vi "Valve_EPICS_Dev4_SSE.vi"() -> ()   [LabVIEW 2014]
uses:
  <userlib>/caLab/Private/Get_PV-1D.vi
  <userlib>/caLab/Private/Put_DBL-1D_PV-1D.vi
panel:
  out "initialized array":i16[](array[numeric])
  in  "stop":bool
  out "sum":i16
  out "0, 1":i16[](array[numeric])
  out "appended array":bool[](array[boolean])
  out "SCL_data":u32[](array[numeric]) caption="data"
  out "SOP_data":u32[](array[numeric]) caption="data"
  out "SCL7":bool
  out "SCL6":bool
  out "SCL5":bool
  out "SCL4":bool
  out "SCL3":bool
  out "SCL2":bool
  out "SCL1":bool
  out "SCL0":bool
  out "SOP7":bool
  out "SOP6":bool
  out "SOP5":bool
  out "SOP4":bool
  out "SOP3":bool
  out "SOP2":bool
  out "SOP1":bool
  out "SOP0":bool
  in  "OPEN7":bool
  in  "OPEN6":bool
  in  "OPEN5":bool
  in  "OPEN4":bool
  in  "OPEN3":bool
  in  "OPEN2":bool
  in  "OPEN1":bool
  in  "OPEN0":bool
  # "Valve control DEV4"
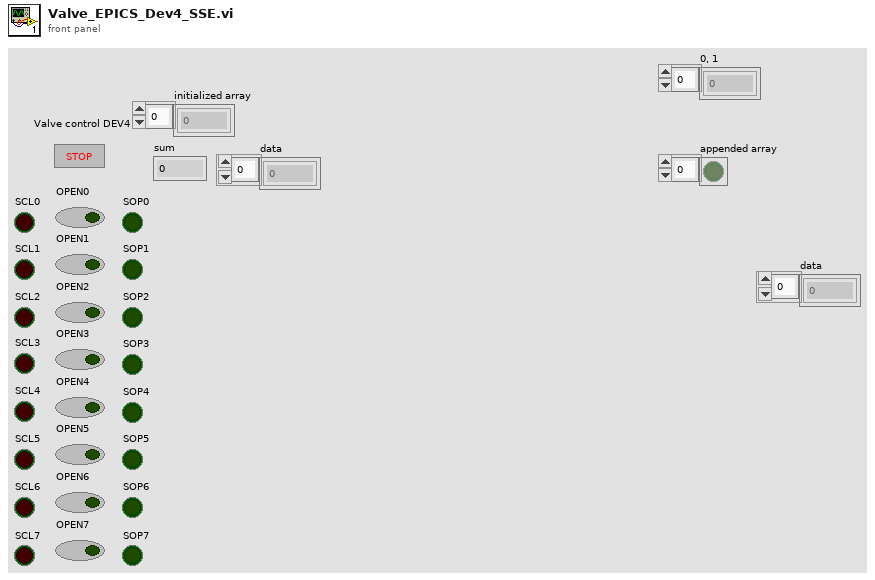
[diagram p1: front panel]
types:
  T1 = typedef "NI_Matrix.lvlib/RealMatrix.ctl" = dbl[][]
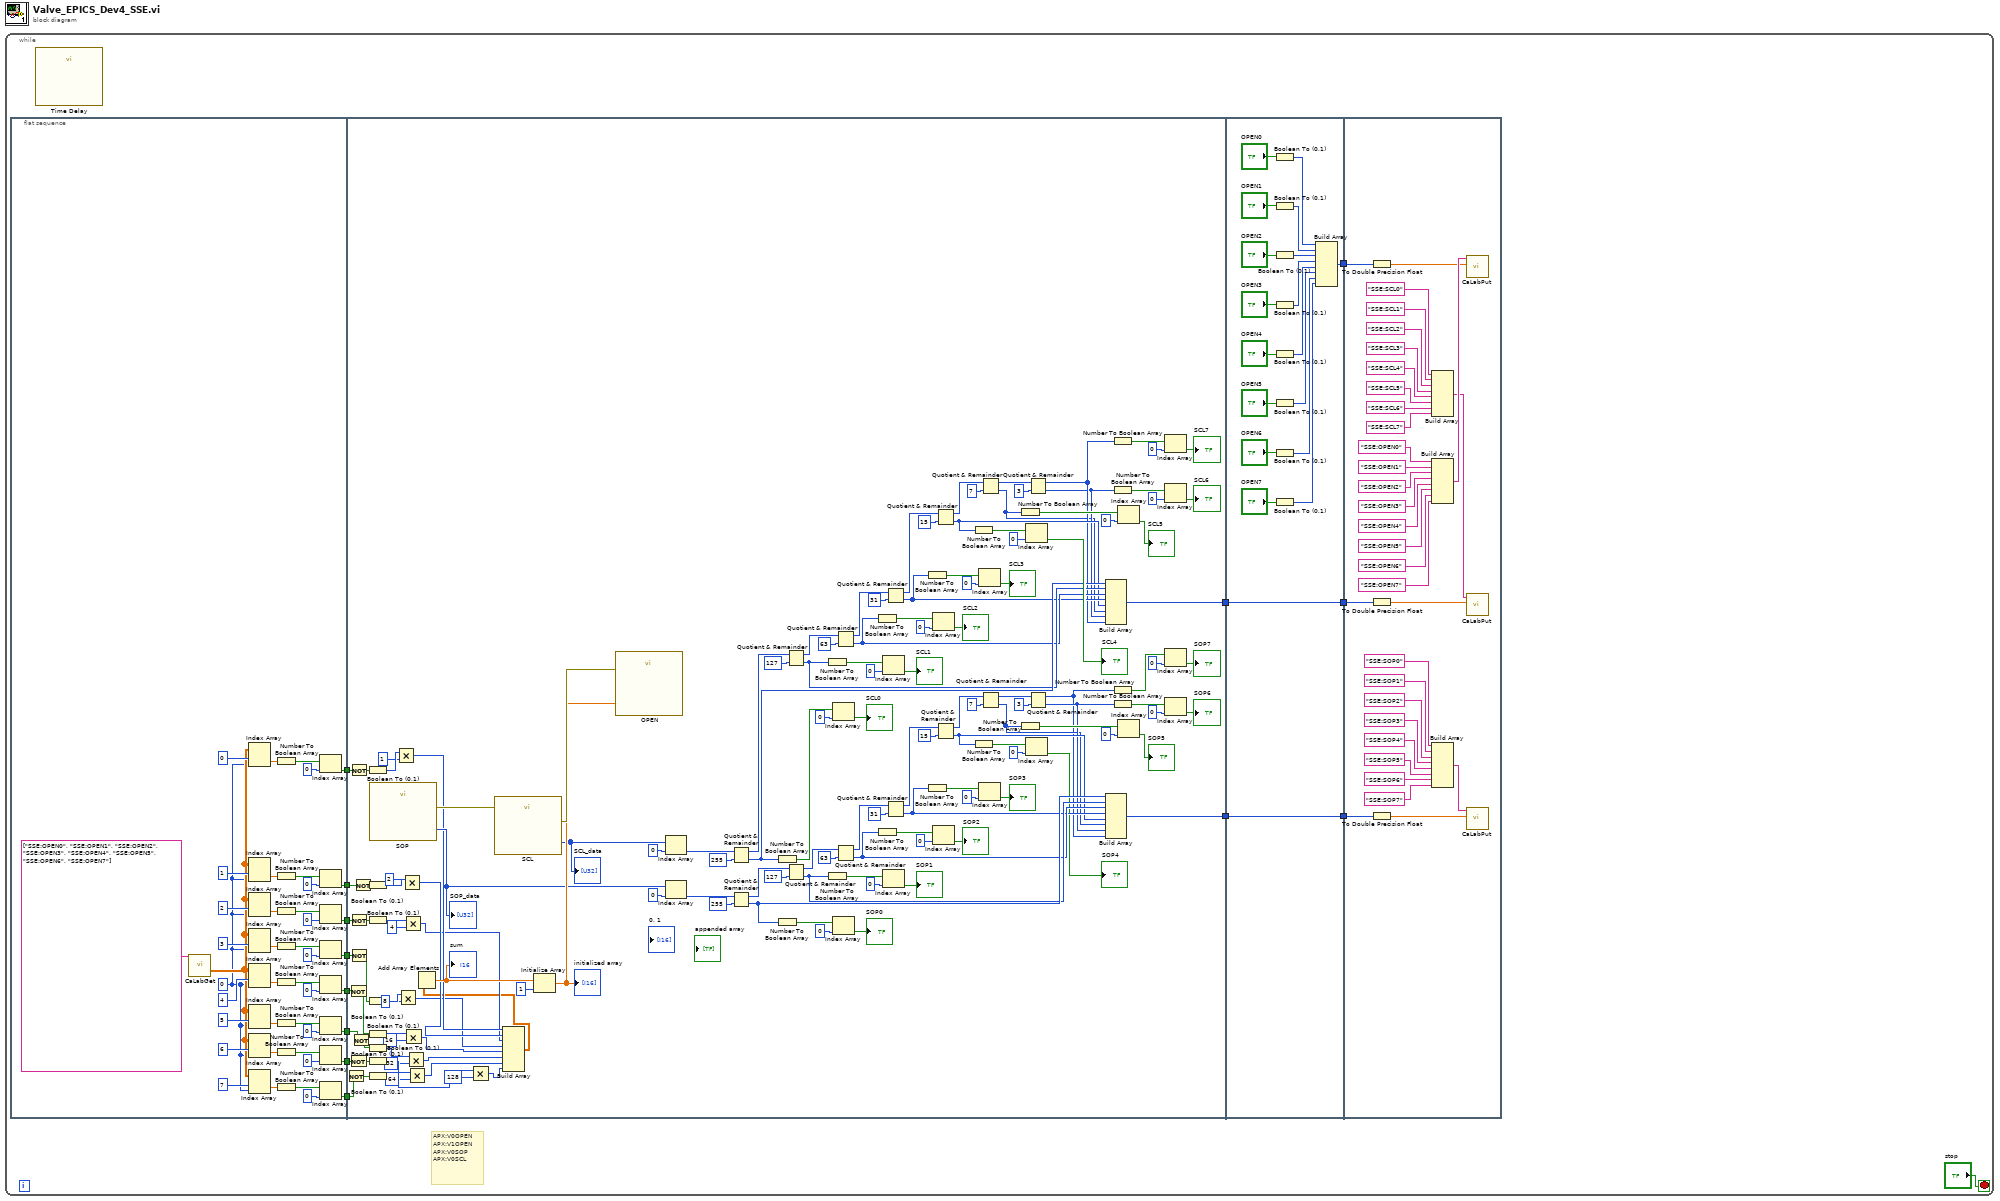
[diagram p0: block diagram]
diagram:
  n1 = while {
    stop <- "stop" stop-if-true
    # "APX:V0OPEN\nAPX:V1OPEN\nAPX:V0SOP\nAPX:V0SCL"
    n2 = flat-sequence {
      tunnel: [w22] -> w14
      tunnel: [w21] -> w13
      tunnel: [w20] -> w12
      tunnel: [w19] -> w11
      tunnel: [w18] -> w10
      tunnel: [w17] -> w9
      tunnel: [w16] -> w8
      tunnel: [w15] -> w7
      tunnel: w14 -> [w174]
      tunnel: w13 -> [w173]
      tunnel: w12 -> [w172]
      tunnel: w11 -> [w171]
      tunnel: w10 -> [w170]
      tunnel: w9 -> [w169]
      tunnel: w8 -> [w168]
      tunnel: w7 -> [w91]
      tunnel: [w141] -> w6
      tunnel: [w92] -> w2
      tunnel: w6 -> [w220]
      tunnel: [w220] -> w5
      tunnel: [w203] -> w4
      tunnel: w2 -> [w202]
      tunnel: [w202] -> w1
      tunnel: w5 -> [w226]
      tunnel: w4 -> [w224]
      tunnel: w1 -> [w222]
      frame #0 {
        w47 = 0 ("index")
        n3 = call-poly "CaLabGet.vi"("PV Names"=string[] ["SSE:OPEN0", "SSE:OPEN1", "SSE:OPEN2", "SSE:OPEN3", "SSE:OPEN4", "SSE:OPEN5", "SSE:OPEN6", "SSE:OPEN7"]) -> ("Value Array (number)"=w48:dbl[][])  [unwired: 8 in, 6 out]
        n4 = Index Array(array=w48, index (row)=0 ("disabled index (row)"), index (col)=w47) -> (element=w27:dbl)
        n5 = Index Array(array=w48, index (row)=1, index (col)=w47) -> (element=w26:dbl)
        n6 = Index Array(array=w48, index (row)=2, index (col)=w47) -> (element=w30:dbl)
        n7 = Index Array(array=w48, index (row)=3 ("index"), index (col)=w47) -> (element=w29:dbl)
        n8 = Index Array(array=w48, index (row)=4, index (col)=w47) -> (element=w28:dbl)
        n9 = Index Array(array=w48, index (row)=5, index (col)=w47) -> (element=w25:dbl)
        n10 = Index Array(array=w48, index (row)=6, index (col)=w47) -> (element=w24:dbl)
        n11 = Index Array(array=w48, index (row)=7, index (col)=w47) -> (element=w23:dbl)
        n12 = Number To Boolean Array(number=w27) -> (Boolean array=w40:bool[])
        n13 = Number To Boolean Array(number=w26) -> (Boolean array=w38:bool[])
        n14 = Number To Boolean Array(number=w30) -> (Boolean array=w46:bool[])
        n15 = Number To Boolean Array(number=w29) -> (Boolean array=w44:bool[])
        n16 = Number To Boolean Array(number=w28) -> (Boolean array=w42:bool[])
        n17 = Number To Boolean Array(number=w25) -> (Boolean array=w36:bool[])
        n18 = Number To Boolean Array(number=w24) -> (Boolean array=w34:bool[])
        n19 = Number To Boolean Array(number=w23) -> (Boolean array=w32:bool[])
        n20 = Index Array(array=w40, index=0) -> (element=w19:bool)
        n21 = Index Array(array=w38, index=0) -> (element=w18:bool)
        n22 = Index Array(array=w46, index=0) -> (element=w22:bool)
        n23 = Index Array(array=w44, index=0) -> (element=w21:bool)
        n24 = Index Array(array=w42, index=0) -> (element=w20:bool)
        n25 = Index Array(array=w36, index=0) -> (element=w17:bool)
        n26 = Index Array(array=w34, index=0) -> (element=w16:bool)
        n27 = Index Array(array=w32, index=0) -> (element=w15:bool)
      }
      frame #1 {
        n28 = Not(x=w91) -> (.not. x?=w75:bool)
        n29 = Not(x=w172) -> (.not. x?=w78:bool)
        n30 = Not(x=w168) -> (.not. x?=w76:bool)
        n31 = Not(x=w171) -> (.not. x?=w82:bool)
        n32 = Not(x=w174) -> (.not. x?=w80:bool)
        n33 = Not(x=w173) -> (.not. x?=w79:bool)
        n34 = Not(x=w169) -> (.not. x?=w77:bool)
        n35 = Not(x=w170) -> (.not. x?=w81:bool)
        n36 = Boolean To (0,1)(Boolean=w82) -> (0, 1=w90:i16)
        n37 = Boolean To (0,1)(Boolean=w81) -> (0, 1=w89:i16)
        n38 = Boolean To (0,1)(Boolean=w80) -> (0, 1=w88:i16)
        n39 = Boolean To (0,1)(Boolean=w79) -> (0, 1=w87:i16)
        n40 = Boolean To (0,1)(Boolean=w78) -> (0, 1=w86:i16)
        n41 = Boolean To (0,1)(Boolean=w77) -> (0, 1=w85:i16)
        n42 = Boolean To (0,1)(Boolean=w76) -> (0, 1=w84:i16)
        n43 = Boolean To (0,1)(Boolean=w75) -> (0, 1=w83:i16)
        n44 = call "SOP"() -> ("data"=w104:u32[], "error out"=w176:errorcluster)  [unwired: 17 in, 1 out]
        "SOP_data" <- w104
        n45 = Multiply(x=w90, y=i16 1) -> (x*y=w66:i16)
        n46 = Multiply(x=w87, y=i16 8) -> (x*y=w63:i16)
        n47 = Multiply(x=w89, y=i16 2) -> (x*y=w65:i16)
        n48 = Multiply(x=w88, y=i16 4) -> (x*y=w64:i16)
        n49 = Multiply(x=w86, y=i16 16) -> (x*y=w62:i16)
        n50 = Multiply(x=w85, y=i16 32) -> (x*y=w61:i16)
        n51 = Multiply(x=w84, y=i16 64) -> (x*y=w60:i16)
        n52 = Multiply(x=w83, y=i16 128) -> (x*y=w59:i16)
        n53 = call "SCL"("error in"=w176) -> ("data"=w164:u32[], "error out"=w175:errorcluster)  [unwired: 16 in, 1 out]
        "SCL_data" <- w164
        n54 = Build Array(w66, w65, w64, w63, w62, w61, w60, w59) -> (w58:T1)
        n55 = Add Array Elements(numeric array=w58) -> (sum=w166:dbl)
        "sum" <- w166
        n56 = Initialize Array(w166, 1 ("dimension size")) -> (w165:dbl[])
        "initialized array" <- w165
        n57 = call "OPEN"("data"=w165, "error in"=w175) -> ()  [unwired: 16 in, 2 out]
        n58 = Index Array(array=w164, index=0) -> (element=w163:u32)
        n59 = Index Array(array=w104, index=0) -> (element=w103:u32)
        n60 = Quotient & Remainder(x=w163, y=u32 255) -> (x-y*floor(x/y)=w161:u32, floor(x/y)=w149:u32)
        n61 = Quotient & Remainder(x=w103, y=u32 255) -> (x-y*floor(x/y)=w124:u32, floor(x/y)=w112:u32)
        n62 = Number To Boolean Array(number=w149) -> (Boolean array=w200:bool[])
        n63 = Number To Boolean Array(number=w112) -> (Boolean array=w140:bool[])
        n64 = Quotient & Remainder(x=w161, y=u32 127) -> (x-y*floor(x/y)=w156:u32, floor(x/y)=w148:u32)
        n65 = Quotient & Remainder(x=w124, y=u32 127) -> (x-y*floor(x/y)=w119:u32, floor(x/y)=w111:u32)
        n66 = Number To Boolean Array(number=w148) -> (Boolean array=w198:bool[])
        n67 = Number To Boolean Array(number=w111) -> (Boolean array=w138:bool[])
        n68 = Index Array(array=w200, index=0) -> (element=→"SCL0":bool)
        n69 = Index Array(array=w140, index=0) -> (element=→"SOP0":bool)
        n70 = Quotient & Remainder(x=w156, y=u32 63) -> (x-y*floor(x/y)=w155:u32, floor(x/y)=w147:u32)
        n71 = Quotient & Remainder(x=w119, y=u32 63) -> (x-y*floor(x/y)=w118:u32, floor(x/y)=w110:u32)
        n72 = Number To Boolean Array(number=w147) -> (Boolean array=w196:bool[])
        n73 = Number To Boolean Array(number=w110) -> (Boolean array=w136:bool[])
        n74 = Index Array(array=w198, index=0) -> (element=→"SCL1":bool)
        n75 = Index Array(array=w138, index=0) -> (element=→"SOP1":bool)
        n76 = Quotient & Remainder(x=w155, y=u32 31) -> (x-y*floor(x/y)=w154:u32, floor(x/y)=w146:u32)
        n77 = Quotient & Remainder(x=w118, y=u32 31) -> (x-y*floor(x/y)=w117:u32, floor(x/y)=w109:u32)
        n78 = Number To Boolean Array(number=w146) -> (Boolean array=w194:bool[])
        n79 = Number To Boolean Array(number=w109) -> (Boolean array=w134:bool[])
        n80 = Index Array(array=w196, index=0) -> (element=→"SCL2":bool)
        n81 = Index Array(array=w136, index=0) -> (element=→"SOP2":bool)
        n82 = Quotient & Remainder(x=w154, y=u32 15) -> (x-y*floor(x/y)=w151:u32, floor(x/y)=w145:u32)
        n83 = Quotient & Remainder(x=w117, y=u32 15) -> (x-y*floor(x/y)=w114:u32, floor(x/y)=w108:u32)
        n84 = Number To Boolean Array(number=w145) -> (Boolean array=w192:bool[])
        n85 = Number To Boolean Array(number=w108) -> (Boolean array=w132:bool[])
        n86 = Index Array(array=w194, index=0) -> (element=→"SCL3":bool)
        n87 = Index Array(array=w134, index=0) -> (element=→"SOP3":bool)
        n88 = Quotient & Remainder(x=w151, y=u32 7) -> (x-y*floor(x/y)=w150:u32, floor(x/y)=w142:u32)
        n89 = Quotient & Remainder(x=w114, y=u32 7) -> (x-y*floor(x/y)=w113:u32, floor(x/y)=w106:u32)
        n90 = Number To Boolean Array(number=w142) -> (Boolean array=w190:bool[])
        n91 = Number To Boolean Array(number=w106) -> (Boolean array=w130:bool[])
        n92 = Index Array(array=w192, index=0) -> (element=→"SCL4":bool)
        n93 = Index Array(array=w132, index=0) -> (element=→"SOP4":bool)
        n94 = Quotient & Remainder(x=w150, y=u32 3) -> (x-y*floor(x/y)=w144:u32, floor(x/y)=w143:u32)
        n95 = Quotient & Remainder(x=w113, y=u32 3) -> (x-y*floor(x/y)=w96:u32, floor(x/y)=w107:u32)
        n96 = Build Array(w149, w148, w147, w146, w145, w142, w143, w144) -> (w141:u32[])
        n97 = Build Array(w112, w111, w110, w109, w108, w106, w107, w96) -> (w92:u32[])
        n98 = Number To Boolean Array(number=w144) -> (Boolean array=w186:bool[])
        n99 = Number To Boolean Array(number=w143) -> (Boolean array=w188:bool[])
        n100 = Number To Boolean Array(number=w96) -> (Boolean array=w95:bool[])
        n101 = Number To Boolean Array(number=w107) -> (Boolean array=w128:bool[])
        n102 = Index Array(array=w190, index=0) -> (element=→"SCL5":bool)
        n103 = Index Array(array=w130, index=0) -> (element=→"SOP5":bool)
        n104 = Index Array(array=w186, index=0) -> (element=→"SCL7":bool)
        n105 = Index Array(array=w188, index=0) -> (element=→"SCL6":bool)
        n106 = Index Array(array=w95, index=0) -> (element=→"SOP7":bool)
        n107 = Index Array(array=w128, index=0) -> (element=→"SOP6":bool)
      }
      frame #2 {
        n108 = Boolean To (0,1)(Boolean="OPEN0") -> (0, 1=w219:i16)
        n109 = Boolean To (0,1)(Boolean="OPEN1") -> (0, 1=w218:i16)
        n110 = Boolean To (0,1)(Boolean="OPEN2") -> (0, 1=w217:i16)
        n111 = Boolean To (0,1)(Boolean="OPEN3") -> (0, 1=w216:i16)
        n112 = Boolean To (0,1)(Boolean="OPEN4") -> (0, 1=w215:i16)
        n113 = Boolean To (0,1)(Boolean="OPEN5") -> (0, 1=w214:i16)
        n114 = Boolean To (0,1)(Boolean="OPEN6") -> (0, 1=w213:i16)
        n115 = Boolean To (0,1)(Boolean="OPEN7") -> (0, 1=w212:i16)
        n116 = Build Array(w219, w218, w217, w216, w215, w214, w213, w212) -> (w203:i16[])
      }
      frame #3 {
        n117 = To Double Precision Float(number=w224) -> (double precision float=w223:dbl[])
        n118 = To Double Precision Float(number=w226) -> (double precision float=w225:dbl[])
        n119 = To Double Precision Float(number=w222) -> (double precision float=w227:dbl[])
        n120 = Build Array("SSE:SCL0", "SSE:SCL1", "SSE:SCL2", "SSE:SCL3", "SSE:SCL4", "SSE:SCL5", "SSE:SCL6", "SSE:SCL7") -> (w228:string[])
        n121 = Build Array("SSE:OPEN0", "SSE:OPEN1", "SSE:OPEN2", "SSE:OPEN3", "SSE:OPEN4", "SSE:OPEN5", "SSE:OPEN6", "SSE:OPEN7") -> (w229:string[])
        n122 = Build Array("SSE:SOP0", "SSE:SOP1", "SSE:SOP2", "SSE:SOP3", "SSE:SOP4", "SSE:SOP5", "SSE:SOP6", "SSE:SOP7") -> (w221:string[])
        n123 = call-poly <userlib>:"CaLabPut.vi"("Values"=w223, "PV Names"=w229) -> ()  [unwired: 6 in, 4 out]
        n124 = call-poly <userlib>:"CaLabPut.vi"("Values"=w225, "PV Names"=w228) -> ()  [unwired: 6 in, 4 out]
        n125 = call-poly <userlib>:"CaLabPut.vi"("Values"=w227, "PV Names"=w221) -> ()  [unwired: 6 in, 4 out]
      }
    }
    n126 = call "Time Delay"() -> ()  [unwired: 11 in, 1 out]
  }
